vi "correctDefenseOutOfField.vi"(6 "Pos Centers Back in":dbl[][](array[numeric]), 8 "error in (no error)":errorcluster, 9 "Number of Defenders\nWithout Duelist":i32, 10 "Game":refnum<class "Game.lvclass">, 11 "Utilities in":refnum<class "Utilities.lvclass">) -> (0 "error out":errorcluster, 2 "Pos Centers Back out":dbl[][](array[numeric]), 3 "Utilities out":refnum<class "Utilities.lvclass">)   [LabVIEW 2023, in "Utilities.lvclass"]
uses:
  Utilities.lvclass
  Game_class/Game.lvclass
  Game_class/Game.lvclass/Game.ctl
  Object_class/Object.lvclass/Object.ctl
  Game_class/Read BallRef.vi
  Game_class/Read FieldRef.vi
  Object_class/Read x.vi
  Object_class/Read y.vi
  Ball_class/Ball.lvclass
  Field_class/Field.lvclass
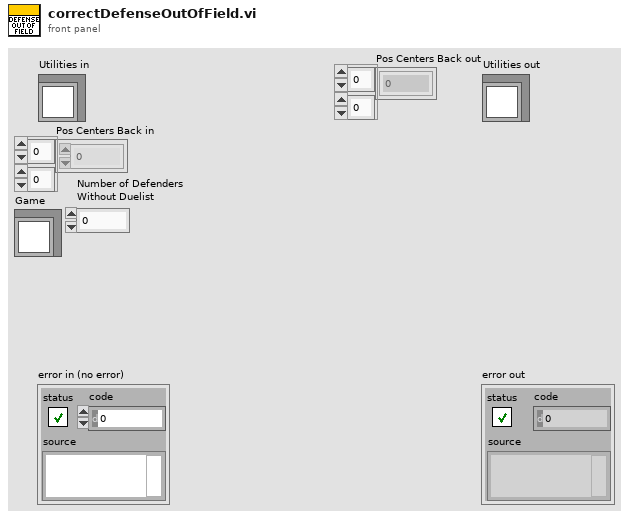
[diagram p1: front panel]
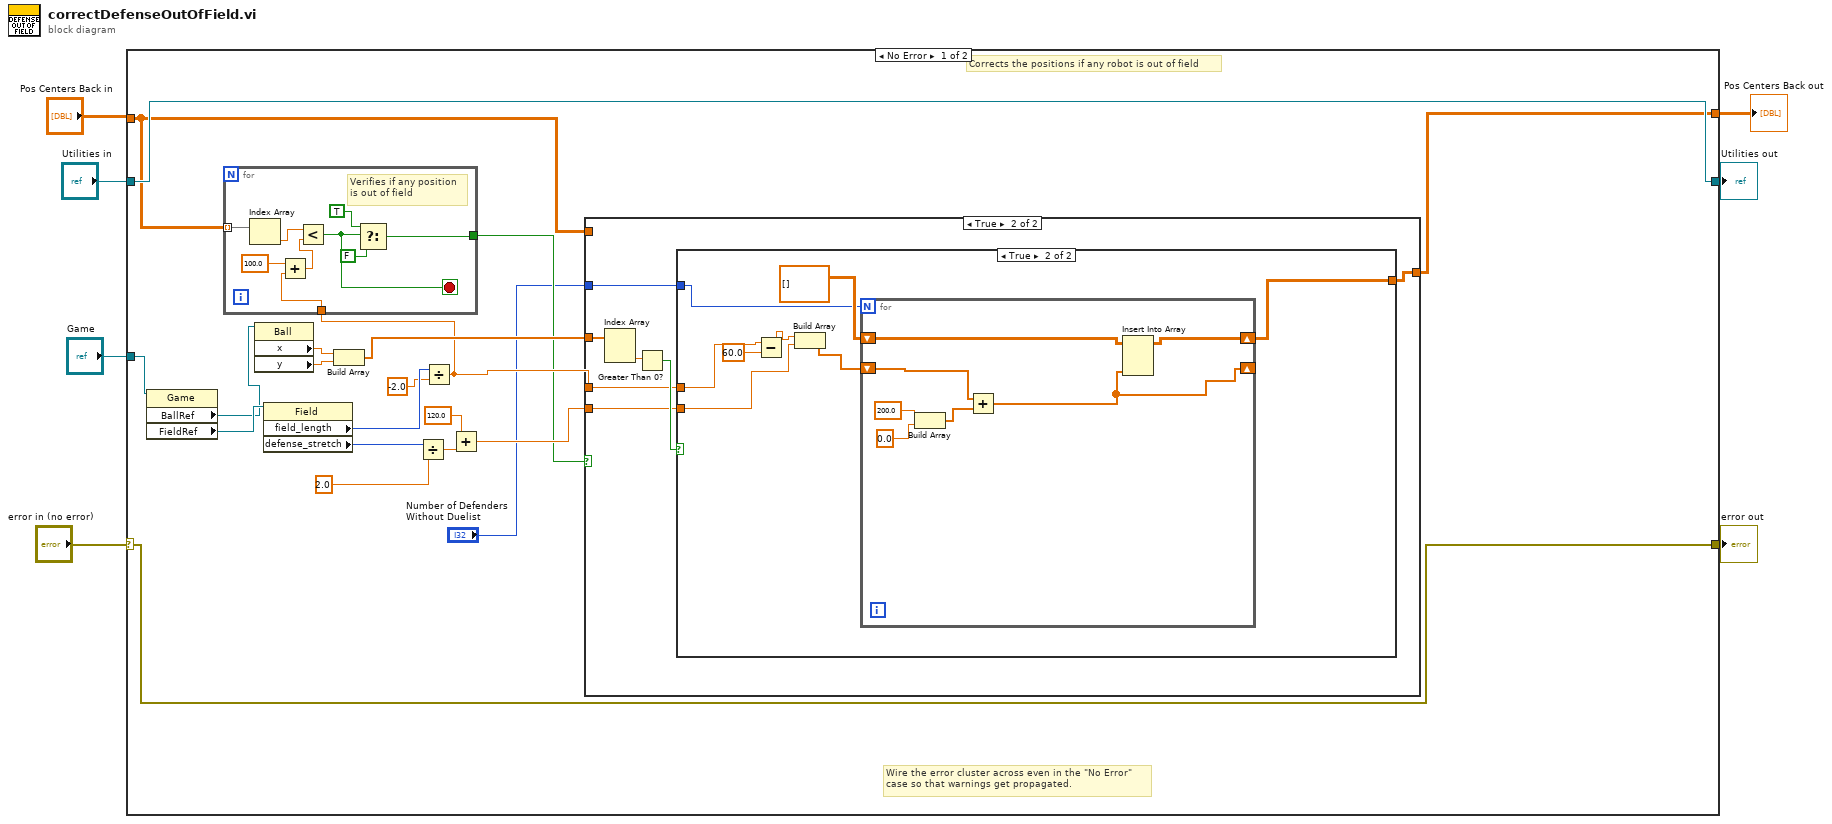
[diagram p0: block diagram]
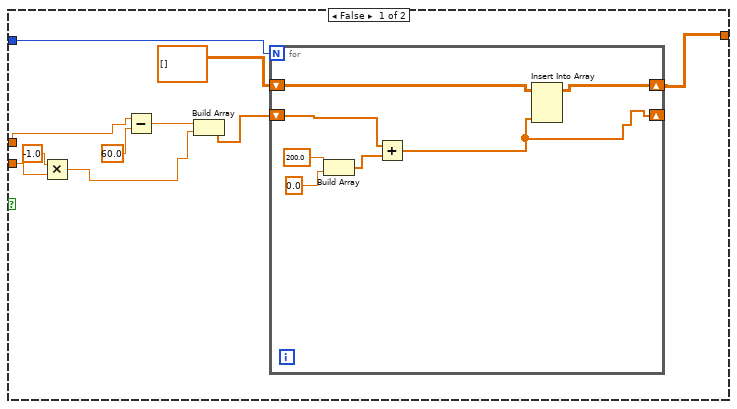
[diagram p3: hidden frame]
diagram:
  n1 = case shown="No Error" "error in (no error)" {
    selector: "error in (no error)" -> [w26 w79]
    tunnel: [w26 w79] -> w6
    tunnel: [w27 w78] -> w4
    tunnel: "Utilities in" -> [w27 w78]
    tunnel: "Game" -> [w25 _]
    tunnel: [w14 w77] -> w2
    tunnel: "Pos Centers Back in" -> [w13 w77]
    frame No Error {
      # "Corrects the positions if any robot is out of field"
      # "Wire the error cluster across even in the \"No Error\"\ncase so that warnings get propagated."
      n2 = property class="Game"(reference=w25) -> ("BallRef"=w18:refnum<class "Ball.lvclass">, "FieldRef"=w24:refnum<class "Field.lvclass">)  [unwired: 1 in, 2 out]
      n3 = property class="Ball"(reference=w18) -> ("x"=w17:dbl, "y"=w16:dbl)  [unwired: 1 in, 2 out]
      n4 = property class="Field"(reference=w24) -> ("field_length"=w9:i32, "defense_stretch"=w23:i32)  [unwired: 1 in, 2 out]
      n5 = Build Array(w17, w16) -> (w15:dbl[])
      n6 = Divide(x=w23, y=2.0) -> (x/y=w21:dbl)
      n7 = Divide(x=w9, y=-2.0) -> (x/y=w12:dbl)
      n8 = for {
        tunnel: w13 -> [w36] mode=indexing
        tunnel: w12 -> [w33]
        tunnel: [w28] -> w11
        stop <- w31 stop-if-true
        # "Verifies if any position\nis out of field"
        n9 = Index Array(array=w36) -> (element=w35:dbl)  [unwired: 1 in]
        n10 = Add(x=100.0, y=w33) -> (x+y=w34:dbl)
        n11 = Less?(x=w35, y=w34) -> (x < y?=w31:bool)
        n12 = Select(t=TRUE, s=w31, f=FALSE) -> (s? t:f=w28:bool)
      }
      n13 = Add(x=120.0, y=w21) -> (x+y=w20:dbl)
      n14 = case shown="True" w11 {
        tunnel: w15 -> [_ w44]
        tunnel: [w37 w40] -> w14
        tunnel: w13 -> [w37 _]
        tunnel: w12 -> [_ w41]
        tunnel: w20 -> [_ w39]
        tunnel: "Number of Defenders\nWithout Duelist" -> [_ w38]
        frame False {
        }
        frame True {
          n15 = Index Array(array=w44) -> (element #2=w43:dbl)  [unwired: 2 in, 1 out]
          n16 = Greater Than 0?(x=w43) -> (x > 0?=w42:bool)
          n17 = case shown="True" w42 {
            tunnel: w41 -> [w53 w68]
            tunnel: [w46 w63] -> w40
            tunnel: w39 -> [w49 w65]
            tunnel: w38 -> [w45 w62]
            frame False {
              n18 = Multiply(x=-1.0, y=w49) -> (x*y=w50:dbl)
              n19 = Subtract(x=w53, y=60.0) -> (x-y=w51:dbl)
              n20 = Build Array(w51, w50) -> (w54:dbl[])
              n21 = for {
                N: w45 -> [_]
                shift-right: [w56] -> w46
                shift-left: dbl[][] [] -> [w57]
                shift-right: [w55] -> _
                shift-left: w54 -> [w58]
                n22 = Build Array(200.0, 0.0) -> (w59:dbl[])
                n23 = Add(x=w58, y=w59) -> (x+y=w55:dbl[])
                n24 = Insert Into Array(array=w57, new element=w55) -> (w56:dbl[][])  [unwired: 2 in]
              }
            }
            frame True {
              n25 = Subtract(x=w68, y=60.0) -> (x-y=w66:dbl)
              n26 = Build Array(w66, w65) -> (w69:dbl[])
              n27 = for {
                N: w62 -> [_]
                shift-right: [w71] -> w63
                shift-left: dbl[][] [] -> [w72]
                shift-right: [w70] -> _
                shift-left: w69 -> [w73]
                n28 = Build Array(200.0, 0.0) -> (w74:dbl[])
                n29 = Add(x=w73, y=w74) -> (x+y=w70:dbl[])
                n30 = Insert Into Array(array=w72, new element=w70) -> (w71:dbl[][])  [unwired: 2 in]
              }
            }
          }
        }
      }
    }
    frame Error {
    }
  }
  "error out" <- w6
  "Utilities out" <- w4
  "Pos Centers Back out" <- w2
